vi "winpcap-llv-mod.vi"() -> ()   [LabVIEW 2020]
panel:
  out "Write Error":bool
  in  "Write Data":bool
  in  "Data to Write":string
  out "Good Read":bool
  out "Timeout":bool
  out "Pkt Len":i32
  out "Pkt uSec":i32
  out "Pkt Sec":i32
  out "Read Error":bool
  in  "Begin Reading Data":bool
  out "Packet Data:":string
  in  "Release All Devices":bool
  out "Error:\nOpen Failed":bool
  in  "Open Device":bool
  out "Error: \nInvalid Device":bool
  out "Opened":bool
  in  "Select Device":u32=1 min=1 max=5 step=1
  out "String 5":string
  out "String 4":string
  out "String 3":string
  out "String 2":string
  out "String":string
  in  "Find Devices":bool
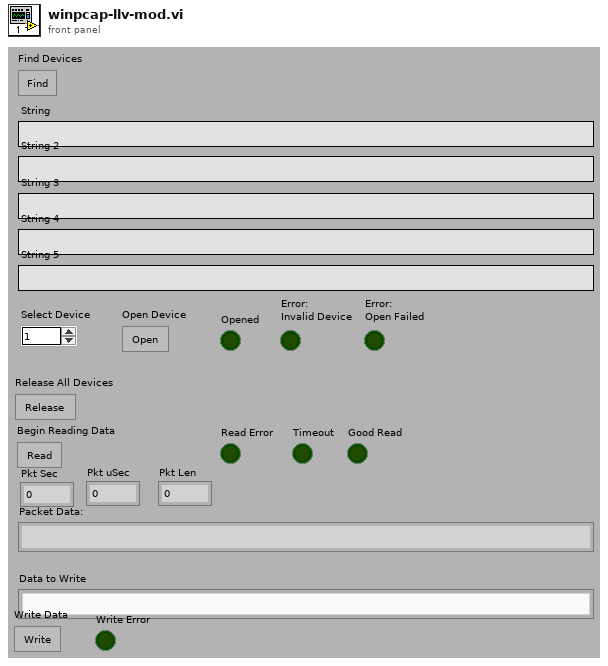
[diagram p1: front panel]
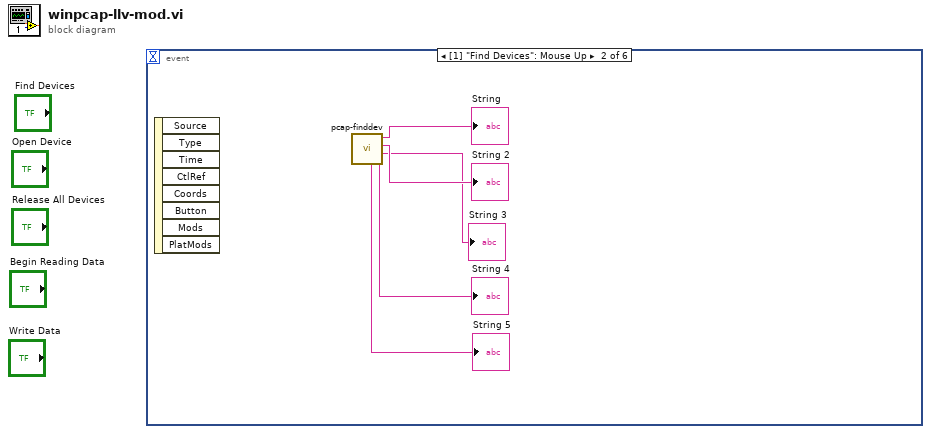
[diagram p0: block diagram]
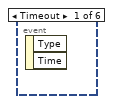
[diagram p2: hidden frame]
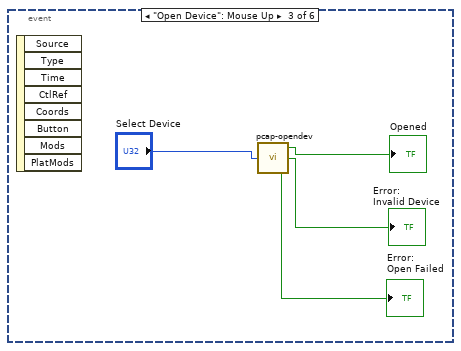
[diagram p3: hidden frame]
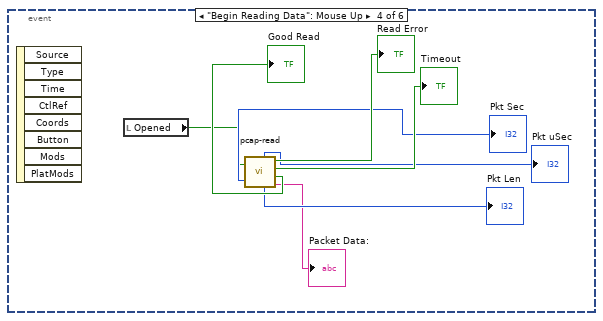
[diagram p4: hidden frame]
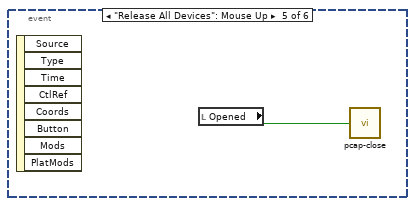
[diagram p5: hidden frame]
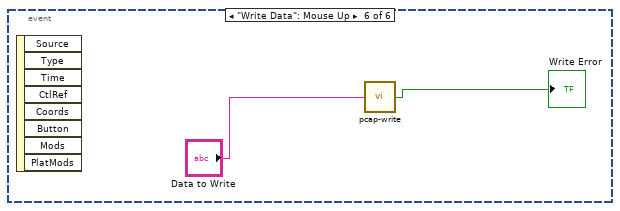
[diagram p6: hidden frame]
diagram:
  n1 = event shown="[1] \"Find Devices\": Mouse Up" {
    selector: _ -> [_ _ _ _ _ _]
    dyn-events: _ -> [_ _ _ _ _ _]
    timeout: _ -> [_ _ _ _ _ _]
    event Timeout {
      n2 = event-data() -> ()  [unwired: 1 in, 2 out]
    }
    event "Find Devices": Mouse Up {
      n3 = event-data() -> ()  [unwired: 1 in, 8 out]
      n4 = call "pcap-finddev.vi"() -> ("String 4"=→"String 4":string, "String 3"=→"String 3":string, "String 2"=→"String 2":string, "String"=→"String":string, "String 5"=→"String 5":string)  [unwired: 1 in]
    }
    event "Open Device": Mouse Up {
      n5 = event-data() -> ()  [unwired: 1 in, 8 out]
      n6 = call "pcap-opendev.vi"("Select Device"="Select Device") -> ("Opened"=→"Opened":bool, "Error: \nInvalid Device"=→"Error: \nInvalid Device":bool, "Error:\nOpen Failed"=→"Error:\nOpen Failed":bool)
    }
    event "Begin Reading Data": Mouse Up {
      n7 = event-data() -> ()  [unwired: 1 in, 8 out]
      n8 = local read "Opened"() -> (w10:bool)
      n9 = call "pcap-read.vi"("Opened"=w10) -> ("Pkt Sec"=→"Pkt Sec":i32, "Pkt uSec"=→"Pkt uSec":i32, "Pkt Len"=→"Pkt Len":i32, "Read Error"=→"Read Error":bool, "Timeout"=→"Timeout":bool, "Good Read"=→"Good Read":bool, "Packet Data:"=→"Packet Data:":string)
    }
    event "Release All Devices": Mouse Up {
      n10 = event-data() -> ()  [unwired: 1 in, 8 out]
      n11 = local read "Opened"() -> (w18:bool)
      n12 = call "pcap-close.vi"("Opened"=w18) -> ()
    }
    event "Write Data": Mouse Up {
      n13 = event-data() -> ()  [unwired: 1 in, 8 out]
      n14 = call "pcap-write.vi"("Data to Write"="Data to Write") -> ("Write Error"=→"Write Error":bool)
    }
  }
